vi "Append Column Headers to Report.vi"(0 "report in":refnum<class "NI_report.lvclass">, 5 "initial header":string, 9 "column headers":string[](array[string]), 11 "error in (no error)":errorcluster) -> (4 "report out":refnum<class "NI_report.lvclass">, 15 "error out":errorcluster)   [LabVIEW 2017, in "NI_ReportGenerationCore.lvlib"]
doc: "Appends array of strings as column headers by placing tabs between them. Called from Append Numeric/Text Table to Report."
uses:
  <vilib>/Utility/NIReport.llb/NI_ReportGenerationCore.lvlib
  <vilib>/Utility/NIReport.llb/NI_report.lvclass
  <vilib>/Utility/NIReport.llb/Append Report Text (str wrap).vi
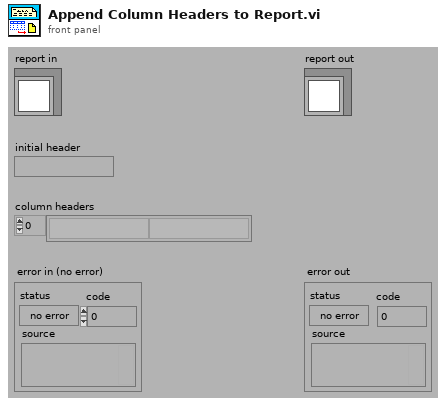
[diagram p1: front panel]
types:
  T1 = cluster{"Italic":enum16{"Italic Unchanged", "Italic On", "Italic Off"}, "Strike Through":enum16{"Strike Through Unchanged", "Strike Through On", "Strike Through Off"}, "Underline":enum16{"Underline Unchanged", "Underline On", "Underline Off"}, "Bold":enum16{"Bold Unchanged", "Bold On", "Bold Off"}}
  T2 = cluster{"Italic":bool, "StrikeThrough":bool, "Underline":bool, "Bold":bool}
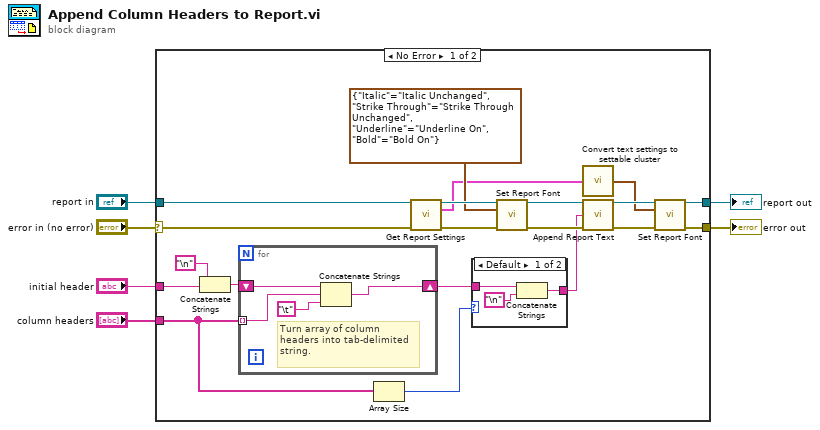
[diagram p0: block diagram]
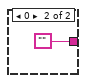
[diagram p2: hidden frame]
diagram:
  n1 = case shown="No Error" "error in (no error)" {
    selector: "error in (no error)" -> [w8 w36]
    tunnel: "column headers" -> [w25 _]
    tunnel: "initial header" -> [w23 _]
    tunnel: [w15 w36] -> w4
    tunnel: [w10 w35] -> w3
    tunnel: "report in" -> [w9 w35]
    frame No Error {
      n2 = Concatenate Strings("\n", w23) -> (w22:string)
      n3 = for {
        tunnel: w25 -> [w33] mode=indexing
        shift-right: [w31] -> w26
        shift-left: w22 -> [w34]
        # "Turn array of column\nheaders into tab-delimited\nstring."
        n4 = Concatenate Strings(w34, w33, "\t") -> (w31:string)
      }
      n5 = Array Size(array=w25) -> (size(s)=w7:i32)
      n6 = call-dynamic "Get Report Settings.vi"("report in"=w9, "error in (no error)"=w8) -> ("report out"=w21:refnum<class "NI_report.lvclass">, "text options"=w12:T2, "error out"=w20:errorcluster)  [unwired: 9 in, 2 out]
      n7 = case shown="Default" w7 {
        tunnel: w26 -> [w29 _]
        tunnel: [w27 ""] -> w14
        frame Default {
          n8 = Concatenate Strings(w29, "\n") -> (w27:string)
        }
        frame 0 {
        }
      }
      n9 = call-dynamic "Set Report Font.vi"("report in"=w21, "text options"=T1 {"Italic"=enum."Italic Unchanged", "Strike Through"=enum."Strike Through Unchanged", "Underline"=enum."Underline On", "Bold"=enum."Bold On"} ("Text Options"), "error in (no error)"=w20) -> ("report out"=w19:refnum<class "NI_report.lvclass">, "error out"=w17:errorcluster)  [unwired: 10 in, 1 out]
      n10 = call <vilib>:"Convert text settings to settable cluster.vi"("cluster from Get Settings"=w12) -> ("cluster for Set Font"=w11:T1)
      n11 = call-poly <vilib>:"Append Report Text.vi"("report in"=w19, "text"=w14, "error in (no error)"=w17) -> ("report out"=w18:refnum<class "NI_report.lvclass">, "error out"=w16:errorcluster)  [unwired: 9 in, 2 out]
      n12 = call-dynamic "Set Report Font.vi"("report in"=w18, "text options"=w11, "error in (no error)"=w16) -> ("report out"=w10:refnum<class "NI_report.lvclass">, "error out"=w15:errorcluster)  [unwired: 10 in, 1 out]
    }
    frame Error {
    }
  }
  "error out" <- w4
  "report out" <- w3
